vi "ModeFieldOriented.vi"() -> (0 "Orientation Mode":T1(ring))   [LabVIEW 2020]
doc: "This VI manages whether the swerve drive is in robot-oriented or field-oriented mode, based on driver inputs, emergency overrides, and safety interlocks."
uses:
  sensordata.vi
  GlobalDrivebase.vi
  GlobalMiscellaneous.vi
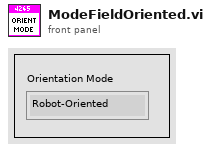
[diagram p1: front panel]
types:
  T1 = enum16{"Robot-Oriented", "Field-Oriented", "Intake"}
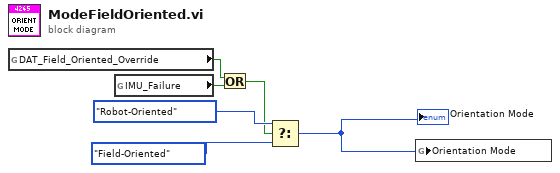
[diagram p0: block diagram]
diagram:
  n1 = global read "GlobalDrivebase.vi" "DAT_Field_Oriented_Override"() -> (w1:bool)
  n2 = global read "sensordata.vi" "IMU_Failure"() -> (w5:bool)
  n3 = Or(x=w1, y=w5) -> (x .or. y?=w4:bool)
  n4 = Select(t=T1."Robot-Oriented", s=w4, f=T1."Field-Oriented") -> (s? t:f=w2:T1)
  "Orientation Mode" <- w2
  n5 = global write "GlobalMiscellaneous.vi" "Orientation Mode"(w2) -> ()
